vi "sunshade color print.vi"(9 "custom number":string, 11 "part type":string) -> (1 "Inalfa Part Number":string, 3 "sunshade color":string)   [LabVIEW 2018]
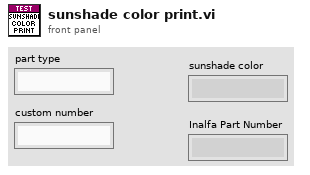
[diagram p1: front panel]
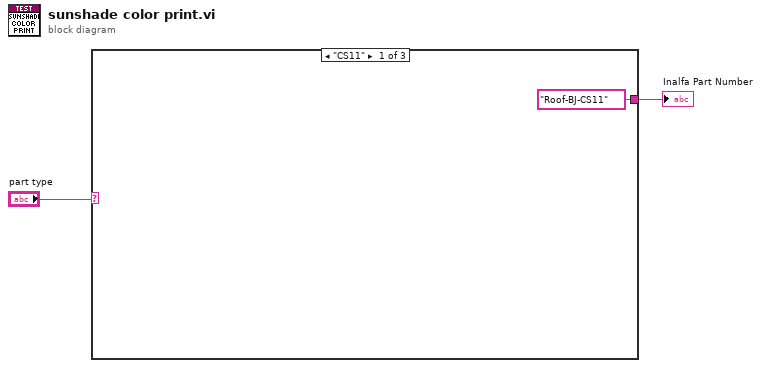
[diagram p0: block diagram]
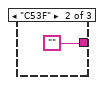
[diagram p2: hidden frame]
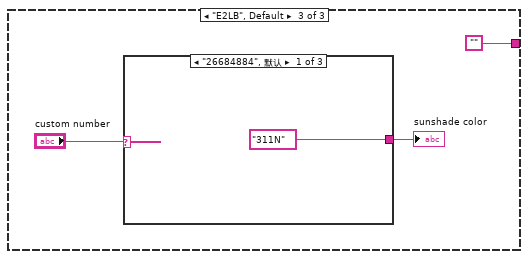
[diagram p3: hidden frame]
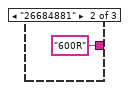
[diagram p4: hidden frame]
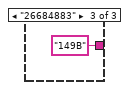
[diagram p5: hidden frame]
diagram:
  n1 = case shown="\"CS11\"" "part type" {
    tunnel: ["Roof-BJ-CS11" "" ""] -> w1
    frame "CS11" {
    }
    frame "C53F" {
    }
    frame "E2LB", Default {
      n2 = case shown="\"26684884\", 默认" "custom number" {
        tunnel: ["311N" ("sunshade color") "600R" ("sunshade color") "149B" ("sunshade color")] -> w6
        frame "26684884", Default {
        }
        frame "26684881" {
        }
        frame "26684883" {
        }
      }
      "sunshade color" <- w6
    }
  }
  "Inalfa Part Number" <- w1
